vi "fit_predict.vi"(8 "error in (no error)":errorcluster, 11 "Interface_fit_predict in":refnum<class "Interface_fit_predict.lvclass">) -> (0 "error out":errorcluster, 2 "labels":dbl[][](array[numeric]), 3 "Interface_fit_predict out":refnum<class "Interface_fit_predict.lvclass">)   [LabVIEW 2020, in "Interface_fit_predict.lvclass"]
doc: "Fit and predict according to the data."
uses:
  Interface_fit_predict.lvclass
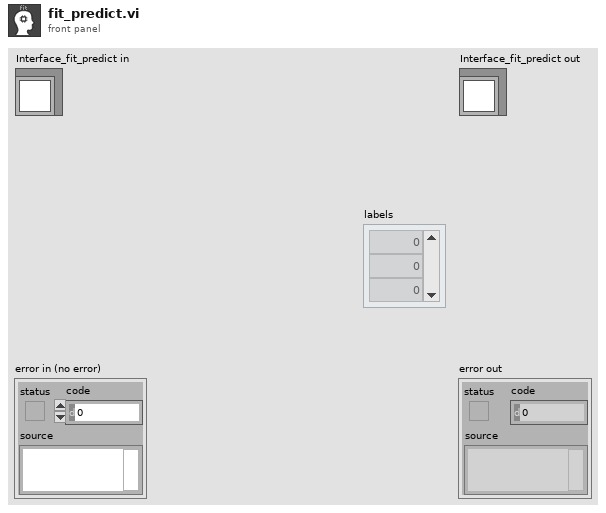
[diagram p1: front panel]
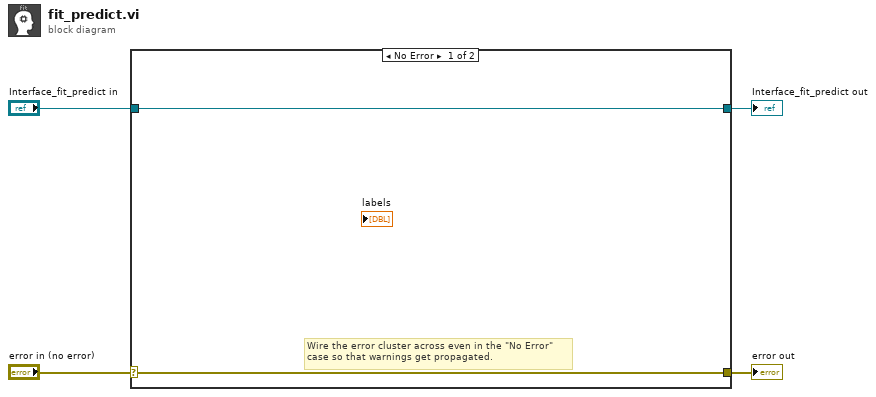
[diagram p0: block diagram]
diagram:
  n1 = case shown="No Error" "error in (no error)" {
    selector: "error in (no error)" -> [w5 w8]
    tunnel: [w5 w8] -> w3
    tunnel: [w6 w7] -> w1
    tunnel: "Interface_fit_predict in" -> [w6 w7]
    frame No Error {
      # "Wire the error cluster across even in the \"No Error\"\ncase so that warnings get propagated."
    }
    frame Error {
    }
  }
  "error out" <- w3
  "Interface_fit_predict out" <- w1
